vi "Wait.Gui.Example.vi"   [LabVIEW 2014]
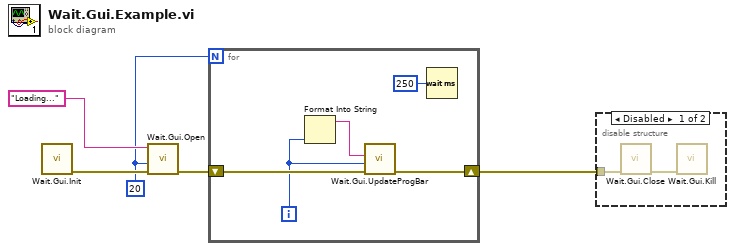
[diagram p0: block diagram]
diagram:
  w1 = 20 ("ProgBarSize (0)")
  n1 = call "Wait.Gui.Init.vi"() -> ("error out"=w5:errorcluster)  [unwired: 11 in]
  n2 = call "Wait.Gui.Open.vi"("error in (no error)"=w5, "ProgBarSize (0)"=w1, "Msg"="Loading...") -> ("error out"=w3:errorcluster)  [unwired: 8 in]
  n3 = for {
    N: w1 -> [_]
    shift-right: [w9] -> w2
    shift-left: w3 -> [w10]
    i -> [w8]
    n4 = Format Into String(w8) -> (resulting string=w7:string)  [unwired: 3 in, 1 out]
    n5 = call "Wait.Gui.UpdateProgBar.vi"("error in (no error)"=w10, "ProgBar (0)"=w8, "status (\"\")"=w7) -> ("error out"=w9:errorcluster)  [unwired: 8 in]
    n6 = Wait (ms)(milliseconds to wait=u32 250) -> ()  [unwired: 1 out]
  }
  n7 = disable-structure shown="Disabled" {
    disable-tunnel: w2 -> [w12 _]
    frame Disabled {
      n8 = call "Wait.Gui.Close.vi"("error in (no error)"=w12) -> ("error out"=w11:errorcluster)  [unwired: 10 in]
      n9 = call "Wait.Gui.Kill.vi"("error in (no error)"=w11) -> ()  [unwired: 10 in, 1 out]
    }
    frame Enabled {
    }
  }
